vi "Add Annotation.vi"(8 "error in (no error)":errorcluster, 9 "Style":T1, 10 "Name":string, 11 "FSM in":refnum<class "FSM.Graph.lvclass">) -> (0 "error out":errorcluster, 2 "Changed?":bool, 3 "FSM out":refnum<class "FSM.Graph.lvclass">)   [LabVIEW 2015, in "FSM.Graph.lvclass"]
uses:
  FSM.Graph.lvclass
  FSM.Annotation/Annotation Style.ctl
  FSM.Graph.lvclass/FSM.Graph.ctl
  FSM.Edge/FSM.Edge.lvclass
  FSM.Annotation/FSM.Annotation.lvclass
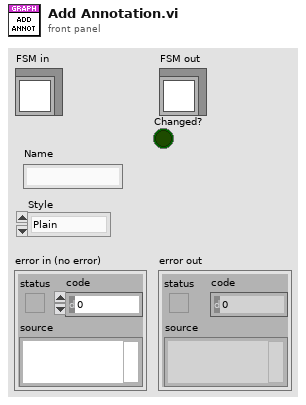
[diagram p1: front panel]
types:
  T1 = typedef "FSM.Annotation.lvclass/Annotation Style.ctl" = enum16{"Plain", "On", "Off", "On-Off"}
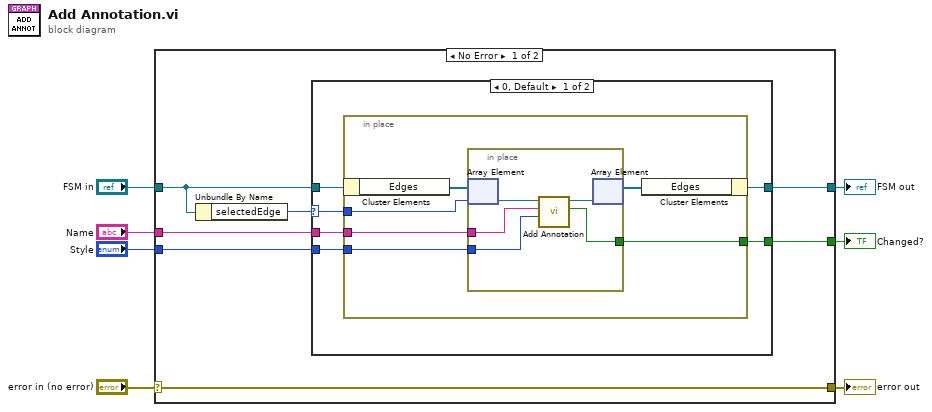
[diagram p0: block diagram]
diagram:
  n1 = case shown="No Error" "error in (no error)" {
    selector: "error in (no error)" -> [w14 w34]
    tunnel: [w14 w34] -> w6
    tunnel: [w11 w33] -> w4
    tunnel: "FSM in" -> [w12 w33]
    tunnel: "Name" -> [w10 _]
    tunnel: "Style" -> [w9 _]
    tunnel: [w8 _] -> w1
    frame No Error {
      n2 = Unbundle By Name(w12) -> ("selectedEdge"=w13:i32)
      n3 = case shown="0, Default" w13 {
        selector: w13 -> [w19 _]
        tunnel: w12 -> [w20 w32]
        tunnel: [w16 w32] -> w11
        tunnel: w10 -> [w18 _]
        tunnel: w9 -> [w17 _]
        tunnel: [w15 _] -> w8
        frame 0, Default {
          n4 = in-place {
            in-place-border: w19 -> [w25]
            in-place-border: w18 -> [w24]
            in-place-border: w17 -> [w23]
            in-place-border: [w21] -> w15
            n5 = in-place-cluster #1(w20) -> ("Edges"=w26:refnum<class "FSM.Edge.lvclass">[])
            n6 = in-place {
              in-place-border: w24 -> [w29]
              in-place-border: w23 -> [w28]
              in-place-border: [w27] -> w21
              n7 = in-place-array #2(w26, w25) -> (w31:refnum<class "FSM.Edge.lvclass">)
              n8 = call "Add Annotation.vi"("Style"=w28, "Name"=w29, "FSM.Edge in"=w31) -> ("Changed?"=w27:bool, "FSM.Edge out"=w30:refnum<class "FSM.Edge.lvclass">)  [unwired: 6 in, 1 out]
              n9 = in-place-array #2(w30) -> (w22:refnum<class "FSM.Edge.lvclass">[])  [unwired: 1 out]
            }
            n10 = in-place-cluster #1("Edges"=w22) -> (w16:refnum<class "FSM.Graph.lvclass">)
          }
        }
        frame -1 {
        }
      }
    }
    frame Error {
    }
  }
  "error out" <- w6
  "FSM out" <- w4
  "Changed?" <- w1
